vi "EventBuilder.destructor.vi"(0 "i ref in":refnum<vi>, 5 "error in (no error)":errorcluster) -> (19 "error out":errorcluster)   [LabVIEW 2014, in "EventBuilder.lvlib"]
doc: "This is the destructor of a class.\n\nLicense Agreement for this software:\n\nCopyright (C)\nGesellschaft für Schwerionenforschung, GSI\nPlanckstr. 1\n64291 Darmstadt\nGermany\n\nContact: D.Beck@gsi.de \n\nThis program is free software; you can redistribute it and/or modify it under the terms of the \nGNU General Public License as published by the Free Software Foundation; either version 2 of \nthe license, or (at your option) any later version.\n\nThis program is distributed in the hope that it will be useful, but WITHOUT ANY WARRANTY; \nwithout even the implied warranty of MERCHANTABILITY or FITNESS FOR A PARTICULAR PURPOSE. See the GNU General License for more details (http://www.gnu.org).\n\nGesellschaft für Schwerionenforschung, GSI\nPlanckstr. 1, 64291 Darmstadt, Germany\nFor all questions and ideas contact: M.Richter@gsi.de, H.Brand@gsi.de or D.Beck@gsi.de.\nLast update: 16-JUN-2004"
uses:
  EventBuilder.lvlib
  CSCore/BaseProcess/BaseProcess.lvlib
  CSlibraries-extern/DimLVEvent/LVDimInterface/LVDimInterface.lvlib
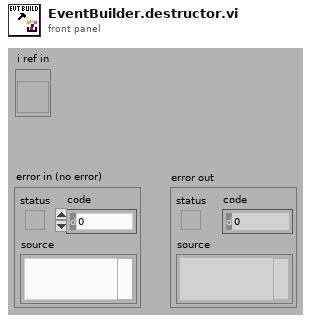
[diagram p1: front panel]
types:
  T1 = typedef "EventBuilder.lvlib/EventBuilder.i attribute.ctl" = cluster{"header":string, "DAQObjs":string[], "headerID":dbl, "eventID":i32, "dataDescriptionID":i32, "eventDataID":i32, "eventDataSize":i32, "dataDescriptionSize":i32}
  T2 = enum16{"SetAttribute", "GetAttribute", "CreateAttribute", "DestroyAttribute", "DestroyAllAtributes"}
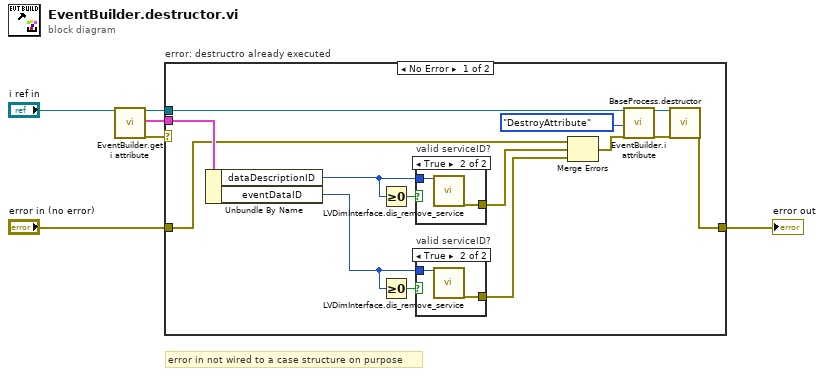
[diagram p0: block diagram]
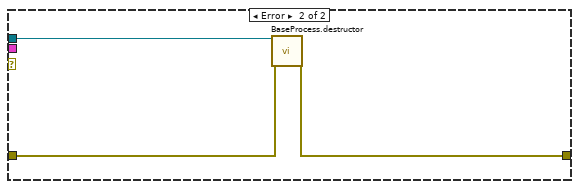
[diagram p4: hidden frame]
diagram:
  # "error in not wired to a case structure on purpose"
  n1 = call "EventBuilder.get i attribute.vi"("i ref in"="i ref in") -> ("i ref out"=w2:refnum<vi>, "i attribute"=w1:T1, "error out"=w3:errorcluster)  [unwired: 16 in]
  n2 = case "error: destructro already executed" shown="No Error" w3 {
    tunnel: [w17 w26] -> w6
    tunnel: "error in (no error)" -> [w11 w25]
    tunnel: w2 -> [w16 w27]
    tunnel: w1 -> [w15 _]
    frame No Error {
      n3 = Unbundle By Name(w15) -> ("dataDescriptionID"=w13:i32, "eventDataID"=w8:i32)
      n4 = Greater Or Equal To 0?(x=w13) -> (x >= 0?=w14:bool)
      n5 = Greater Or Equal To 0?(x=w8) -> (x >= 0?=w9:bool)
      n6 = case "valid serviceID?" shown="True" w14 {
        tunnel: w13 -> [_ w24]
        tunnel: [_ w23] -> w10
        frame False {
        }
        frame True {
          n7 = call "LVDimInterface.dis_remove_service.vi"("my_serviceID"=w24) -> ("error out"=w23:errorcluster)  [unwired: 18 in]
        }
      }
      n8 = case "valid serviceID?" shown="True" w9 {
        tunnel: w8 -> [_ w22]
        tunnel: [_ w21] -> w7
        frame False {
        }
        frame True {
          n9 = call "LVDimInterface.dis_remove_service.vi"("my_serviceID"=w22) -> ("error out"=w21:errorcluster)  [unwired: 18 in]
        }
      }
      n10 = Merge Errors(w11, w10, w7) -> (w12:errorcluster)
      n11 = call "EventBuilder.i attribute.vi"("VI Refnum"=w16, "Action"=T2."DestroyAttribute", "error in (no error)"=w12) -> ("VI Refnum out"=w19:refnum<vi>, "error out"=w18:errorcluster)  [unwired: 14 in, 1 out]
      n12 = call "BaseProcess.destructor.vi"("i ref in"=w19, "error in (no error)"=w18) -> ("error out"=w17:errorcluster)  [unwired: 17 in]
    }
    frame Error {
      n13 = call "BaseProcess.destructor.vi"("i ref in"=w27, "error in (no error)"=w25) -> ("error out"=w26:errorcluster)  [unwired: 17 in]
    }
  }
  "error out" <- w6
